vi "Get Type.vi"(8 "error in (no error)":errorcluster, 11 "Small Register Bank in":refnum<class "Small Register Bank.lvclass">) -> (0 "error out":errorcluster, 2 "Item Type":T1, 3 "Small Register Bank out":refnum<class "Small Register Bank.lvclass">)   [LabVIEW 2020, in "Small Register Bank.lvclass"]
uses:
  Small Register Bank.lvclass
  Item/Item Type.ctl
  Item/Item.lvclass
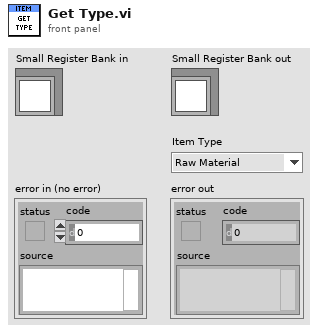
[diagram p1: front panel]
types:
  T1 = typedef "Item.lvclass/Item Type.ctl" = enum16{"Raw Material", "Component", "Module", "Product"}
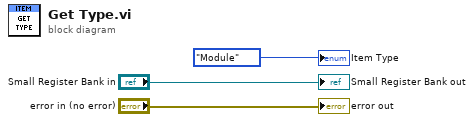
[diagram p0: block diagram]
diagram:
  "error out" <- "error in (no error)"
  "Small Register Bank out" <- "Small Register Bank in"
  "Item Type" <- Item_Type."Module" ("Item Type")
